vi "GEA2 Initialize Multiple Devices.vi"(0 "Source Addresses":u8[](array[numeric]) format="%.0x", 11 "error in":errorcluster) -> (4 "Array of GEA2 References Out":refnum<k24>[](array[refnum]), 8 "Board IDs":string[](array[string]), 15 "error out":errorcluster)   [LabVIEW 2014, in "GEA2_Toolkit.lvlib"]
doc: "This VI uses .NET DLLs to initialize a GEA2 connection over USB to multiple devices. The output is an array of references to the newly opened GEA2 connections."
uses:
  library/GEA2_Toolkit.lvlib
  C:/Automation/DLLs/PC Tools .NET/GeaCommunication.dll
  Automation/DLLs/PC Tools .NET/GeaCommunication.dll
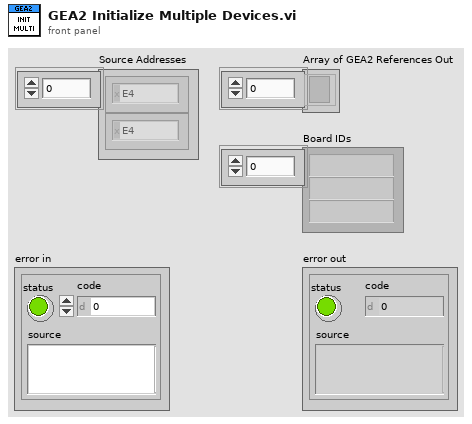
[diagram p1: front panel]
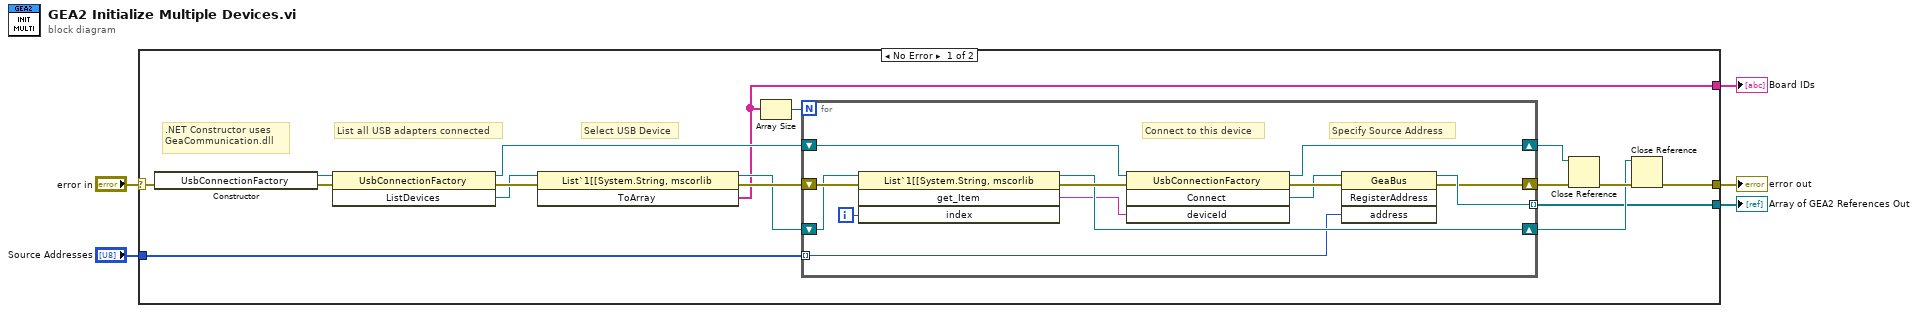
[diagram p0: block diagram]
diagram:
  n1 = case shown="No Error" "error in" {
    selector: "error in" -> [w20 w36]
    tunnel: [w8 w36] -> w5
    tunnel: [w6 _] -> w1
    tunnel: "Source Addresses" -> [w14 _]
    tunnel: [w12 _] -> w2
    frame No Error {
      # "Select USB Device"
      # "List all USB adapters connected"
      # ".NET Constructor uses\nGeaCommunication.dll"
      n2 = constructor class="UsbConnectionFactory"(error in=w20) -> (reference out=w18:refnum<k24>, error out=w19:errorcluster)  [unwired: 2 in, 1 out]
      n3 = invoke class="UsbConnectionFactory" method="ListDevices"(reference=w18, error in=w19) -> (reference out=w17:refnum<k24>, error out=w22:errorcluster, "ListDevices"=w21:refnum<k24>)  [unwired: 1 in]
      n4 = invoke class="List`1[[System.String, mscorlib" method="ToArray"(reference=w21, error in=w22) -> (reference out=w15:refnum<k24>, error out=w16:errorcluster, "ToArray"=w12:string[])  [unwired: 1 in]
      n5 = Array Size(array=w12) -> (size(s)=w13:i32)
      n6 = for {
        N: w13 -> [_]
        tunnel: [w34] -> w6 mode=indexing
        shift-right: [w25] -> w10
        shift-left: w17 -> [w32]
        shift-right: [w24] -> w11
        shift-left: w16 -> [w31]
        shift-right: [w27] -> w7
        shift-left: w15 -> [w29]
        tunnel: w14 -> [w23] mode=indexing
        i -> [w28]
        # "Specify Source Address"
        # "Connect to this device"
        n7 = invoke class="List`1[[System.String, mscorlib" method="get_Item"(reference=w29, error in=w31, "index"=w28) -> (reference out=w27:refnum<k24>, error out=w30:errorcluster, "get_Item"=w26:string)  [unwired: 1 in, 1 out]
        n8 = invoke class="UsbConnectionFactory" method="Connect"(reference=w32, error in=w30, "deviceId"=w26) -> (reference out=w25:refnum<k24>, error out=w35:errorcluster, "Connect"=w33:refnum<k24>)  [unwired: 1 in, 1 out]
        n9 = invoke class="GeaBus" method="RegisterAddress"(reference=w33, error in=w35, "address"=w23) -> (reference out=w34:refnum<k24>, error out=w24:errorcluster)  [unwired: 1 in, 2 out]
      }
      n10 = Close Reference(reference=w10, error in (no error)=w11) -> (error out=w9:errorcluster)
      n11 = Close Reference(reference=w7, error in (no error)=w9) -> (error out=w8:errorcluster)
    }
    frame Error {
    }
  }
  "error out" <- w5
  "Board IDs" <- w2
  "Array of GEA2 References Out" <- w1
